vi "oa_Find Start Speed.vi"(7 "reset":bool, 9 "steps input":cluster{"start":dbl, "end":dbl, "step":dbl} {"step" format="%.2f"; "end" format="%.2f"; "start" format="%.2f"}, 10 "start found":bool, 11 "reference array":dbl[](array[numeric])) -> (2 "find start?":bool)   [LabVIEW 2017]
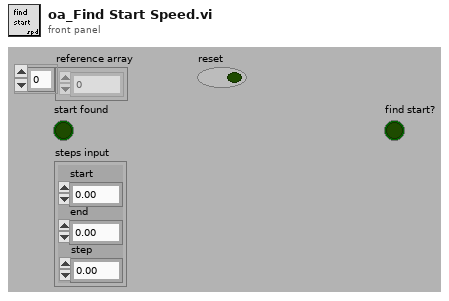
[diagram p1: front panel]
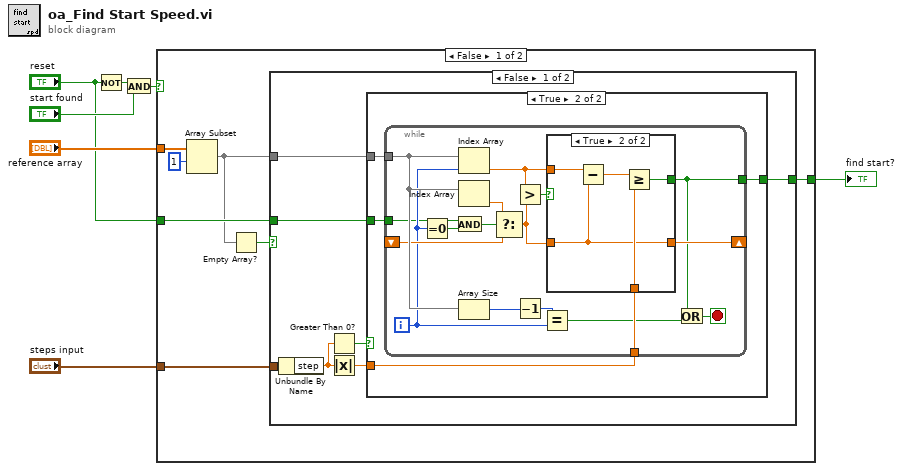
[diagram p0: block diagram]
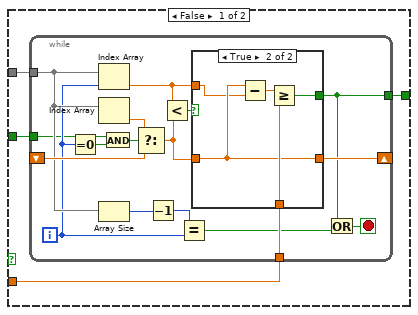
[diagram p2: hidden frame]
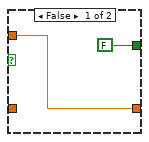
[diagram p3: hidden frame]
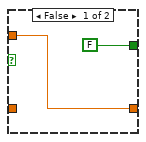
[diagram p4: hidden frame]
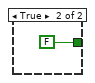
[diagram p5: hidden frame]
diagram:
  n1 = Not(x="reset") -> (.not. x?=w4:bool)
  n2 = And(x=w4, y="start found") -> (x .and. y?=w2:bool)
  n3 = case shown="False" w2 {
    selector: w2 -> [_ w79]
    tunnel: "reference array" -> [w14 _]
    tunnel: [w12 w79] -> w6
    tunnel: "steps input" -> [w13 _]
    tunnel: "reset" -> [w10 _]
    frame False {
      n4 = Array Subset(array=w14, index=1) -> (w9:dbl[])  [unwired: 1 in]
      n5 = Empty Array?(array=w9) -> (empty?=w8:bool)
      n6 = case shown="False" w8 {
        tunnel: w13 -> [w21 _]
        tunnel: [w20 FALSE] -> w12
        tunnel: w9 -> [w16 _]
        tunnel: w10 -> [w15 _]
        frame False {
          n7 = Unbundle By Name(w21) -> ("step"=w18:dbl)
          n8 = Greater Than 0?(x=w18) -> (x > 0?=w17:bool)
          n9 = Absolute Value(x=w18) -> (abs(x)=w19:dbl)
          n10 = case shown="True" w17 {
            tunnel: w16 -> [w25 w53]
            tunnel: w19 -> [w23 w52]
            tunnel: [w22 w51] -> w20
            tunnel: w15 -> [w24 w50]
            frame False {
              n11 = while {
                tunnel: w25 -> [w31]
                shift-right: [w41] -> _
                shift-left: _ -> [w33]
                tunnel: w23 -> [w40]
                tunnel: [w38] -> w22
                tunnel: w24 -> [w27]
                i -> [w29]
                stop <- w36 stop-if-true
                n12 = Equal To 0?(x=w29) -> (x = 0?=w28:bool)
                n13 = Index Array(array=w31, index=w29) -> (element=w35:dbl)
                n14 = Index Array(array=w31) -> (element=w34:dbl)  [unwired: 1 in]
                n15 = Array Size(array=w31) -> (size(s)=w30:i32)
                n16 = And(x=w27, y=w28) -> (x .and. y?=w26:bool)
                n17 = Select(t=w34, s=w26, f=w33) -> (s? t:f=w32:dbl)
                n18 = Decrement(x=w30) -> (x-1=w39:i32)
                n19 = Less?(x=w35, y=w32) -> (x < y?=w42:bool)
                n20 = Equal?(x=w39, y=w29) -> (x = y?=w37:bool)
                n21 = case shown="True" w42 {
                  tunnel: w35 -> [w44 w45]
                  tunnel: [w44 w46] -> w41
                  tunnel: w32 -> [_ w46]
                  tunnel: w40 -> [_ w48]
                  tunnel: [FALSE w47] -> w38
                  frame False {
                  }
                  frame True {
                    n22 = Subtract(x=w46, y=w45) -> (x-y=w49:dbl)
                    n23 = Greater Or Equal?(x=w49, y=w48) -> (x >= y?=w47:bool)
                  }
                }
                n24 = Or(x=w38, y=w37) -> (x .or. y?=w36:bool)
              }
            }
            frame True {
              n25 = while {
                tunnel: w53 -> [w60]
                shift-right: [w69] -> _
                shift-left: _ -> [w58]
                tunnel: w52 -> [w68]
                tunnel: [w66] -> w51
                tunnel: w50 -> [w55]
                i -> [w57]
                stop <- w64 stop-if-true
                n26 = Equal To 0?(x=w57) -> (x = 0?=w56:bool)
                n27 = And(x=w55, y=w56) -> (x .and. y?=w54:bool)
                n28 = Index Array(array=w60, index=w57) -> (element=w63:dbl)
                n29 = Index Array(array=w60) -> (element=w62:dbl)  [unwired: 1 in]
                n30 = Array Size(array=w60) -> (size(s)=w59:i32)
                n31 = Select(t=w62, s=w54, f=w58) -> (s? t:f=w61:dbl)
                n32 = Greater?(x=w63, y=w61) -> (0:w70:bool)
                n33 = Decrement(x=w59) -> (x-1=w67:i32)
                n34 = Equal?(x=w67, y=w57) -> (x = y?=w65:bool)
                n35 = case shown="True" w70 {
                  tunnel: w63 -> [w72 w77]
                  tunnel: [w72 w73] -> w69
                  tunnel: w61 -> [_ w73]
                  tunnel: w68 -> [_ w75]
                  tunnel: [FALSE w74] -> w66
                  frame False {
                  }
                  frame True {
                    n36 = Subtract(x=w77, y=w73) -> (x-y=w76:dbl)
                    n37 = Greater Or Equal?(x=w76, y=w75) -> (x >= y?=w74:bool)
                  }
                }
                n38 = Or(x=w66, y=w65) -> (x .or. y?=w64:bool)
              }
            }
          }
        }
        frame True {
        }
      }
    }
    frame True {
    }
  }
  "find start?" <- w6
